vi "ToDGMLContent.vi"(6 "Export type":T1, 8 "error in (no error)":errorcluster, 9 "Parameters":string, 10 "IReporter":refnum<class "IExporter.lvclass">, 11 "CDependencyList in":refnum<class "CDependencyList.lvclass">) -> (0 "error out":errorcluster, 3 "CDependencyList out":refnum<class "CDependencyList.lvclass">)   [LabVIEW 2020, in "DependencyInspection.lvlib" / "CDependencyList.lvclass"]
uses:
  CDependencyList.lvclass
  obj/Addons/ExtensionInterfaces.lvlibp/IExporter/IExporter.lvclass
  obj/Addons/ExtensionInterfaces.lvlibp/IExporter/ExportType.ctl
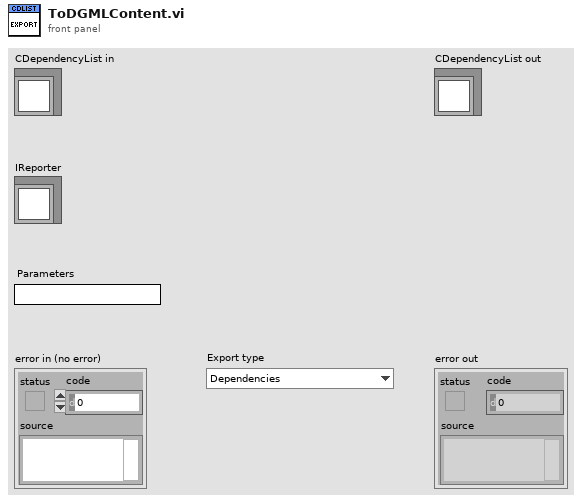
[diagram p1: front panel]
types:
  T1 = typedef "ExtensionInterfaces.lvlibp/IExporter.lvclass/ExportType.ctl" = enum16{"Dependencies", "Rules", "Invalid dependencies", "Concessions", "Undeclared"}
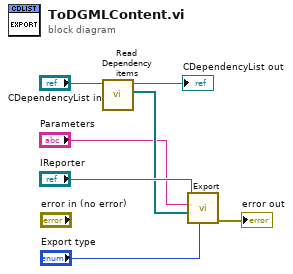
[diagram p0: block diagram]
diagram:
  n1 = call-dynamic "Read Dependency items.vi"("CDependencyList in"="CDependencyList in") -> ("Dependency items"=w4:refnum<class "ILabVIEWItem.lvclass">[], "CDependencyList out"=→"CDependencyList out":refnum<class "CDependencyList.lvclass">)  [unwired: 9 in]
  n2 = call-dynamic "Export.vi"("Export type"="Export type", "Items"=w4, "Parameters"="Parameters", "IExporter in"="IReporter") -> ("error out"=→"error out":errorcluster)  [unwired: 6 in, 1 out]
